vi "Get Last Plot Fit Data.vi"(8 "error in (no error)":errorcluster, 11 "XYGraph in":refnum<vi>) -> (0 "error out":errorcluster, 3 "Last Fit Data":T1)   [LabVIEW 2019, in "Histogram Window.lvlib"]
uses:
  Histogram Window.lvlib
  Plot Histogram.ctl
  Graphs/Plot Style 3.ctl
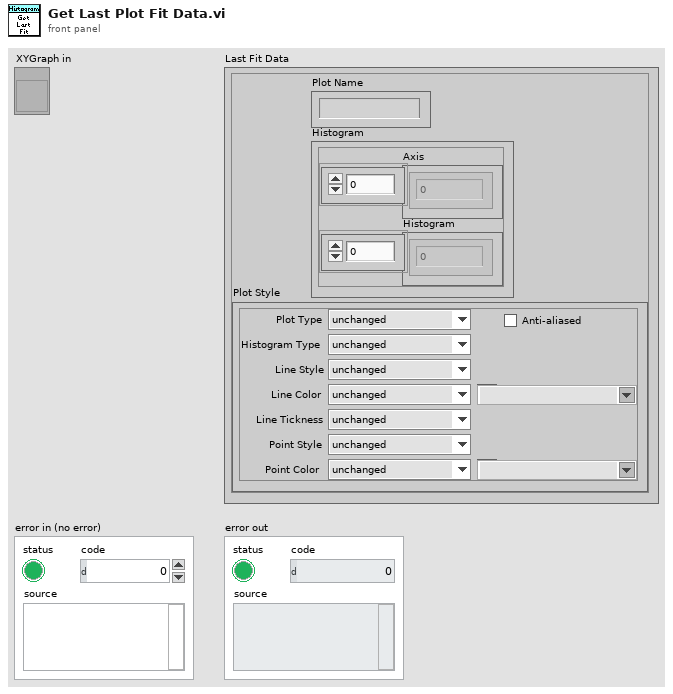
[diagram p1: front panel]
types:
  T1 = typedef "Histogram Window.lvlib/Plot Histogram.ctl" = cluster{"Plot Name":string, "Histogram":cluster{"Axis":dbl[], "Histogram":dbl[]}, "Plot Style":T2}
  T2 = typedef "Plot Style 3.ctl" = cluster{"Plot Style":enum16{"unchanged", "Line", "Symbol", "Line + Symbol", "Histogram", "Histogram + Symbol"}, "Histogram Type":enum16{"unchanged", "Left Bound", "Center", "Right Bound"}, "Line Tickness":enum16{"unchanged", "Thin", "1 pixel", "2 pixel", "3 pixel", "4 pixel", "5 pixel"}, "Line Style":enum16{"unchanged", "Plain", "Long Dash", "Short Dash", "Long-Short Dash", "Long-Short-Short Dash"}, "Point Style":enum16{"unchanged", "None", "Empty Circle", "Filled Circle", "Thick Circle", "Dotted Circle", "Empty Square", "Filled Square", "Thick Square", "Dotted Square", "Small Filled Square", "Dot", "Cross", "Tiny Cross", "Large X", "Small x", "Diamond", "Small Empty Square"}, "Line Color":u32, "Point Color":u32, "Anti-aliased":bool, "Line Color Chooser":enum16{"unchanged", "Color Box", "Color List"}, "Point Color Chooser":enum16{"unchanged", "Color Box", "Color List"}, "Line Color List":string, "Point Color List":string}
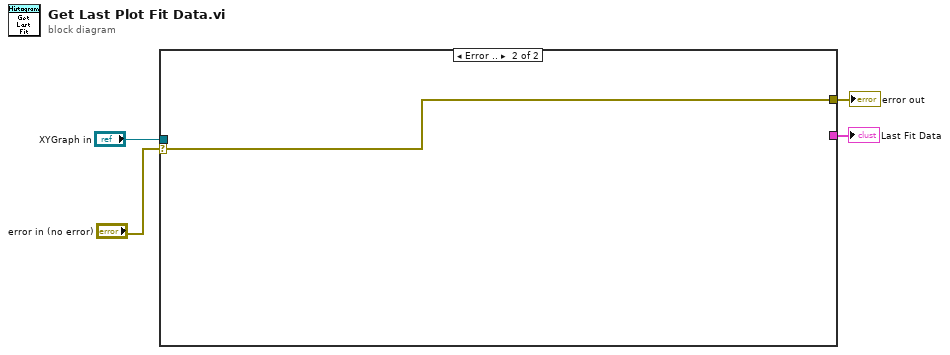
[diagram p0: block diagram]
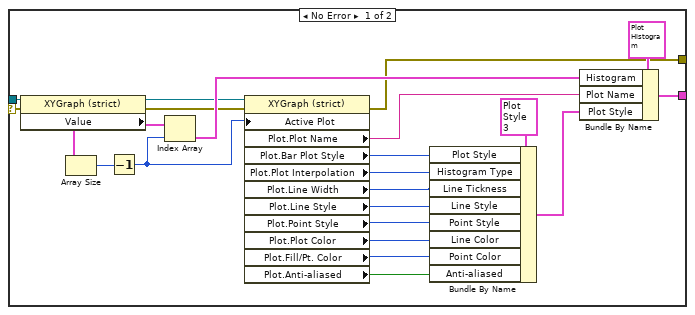
[diagram p2: hidden frame]
diagram:
  n1 = case shown="Error .." "error in (no error)" {
    selector: "error in (no error)" -> [w23 w27]
    tunnel: [w26 _] -> w4
    tunnel: "XYGraph in" -> [w24 _]
    tunnel: [w5 w27] -> w1
    frame No Error {
      n2 = property class="XYGraph (strict)"(reference=w24, error in=w23) -> (reference out=w19:refnum<vi>, error out=w18:errorcluster, "Value"=w22:cluster{"Axis":dbl[], "Histogram":dbl[]}[])
      n3 = Array Size(array=w22) -> (size(s)=w21:i32)
      n4 = Decrement(x=w21) -> (x-1=w17:i32)
      n5 = Index Array(array=w22, index=w17) -> (element=w20:cluster{"Axis":dbl[], "Histogram":dbl[]})
      n6 = property class="XYGraph (strict)"(reference=w19, error in=w18, "Active Plot"=w17) -> (error out=w5:errorcluster, "Plot.Plot Name"=w16:string, "Plot.Bar Plot Style"=w13:u8, "Plot.Plot Interpolation"=w14:u8, "Plot.Line Width"=w12:u8, "Plot.Line Style"=w11:u8, "Plot.Point Style"=w10:u8, "Plot.Plot Color"=w9:u32, "Plot.Fill/Pt. Color"=w8:u32, "Plot.Anti-aliased"=w7:bool)  [unwired: 1 out]
      n7 = Bundle By Name(cluster=T2 {"Plot Style"=enum."unchanged", "Histogram Type"=enum."Left Bound", "Line Tickness"=enum."unchanged", "Line Style"=enum."unchanged", "Point Style"=enum."unchanged", "Line Color"=0, "Point Color"=0, "Anti-aliased"=FALSE, "Line Color Chooser"=enum."unchanged", "Point Color Chooser"=enum."unchanged", "Line Color List"="", "Point Color List"=""} ("Plot Style"), "Plot Style"=w13, "Histogram Type"=w14, "Line Tickness"=w12, "Line Style"=w11, "Point Style"=w10, "Line Color"=w9, "Point Color"=w8, "Anti-aliased"=w7) -> (w6:T2)
      n8 = Bundle By Name(cluster=T1 {"Plot Name"="", "Histogram"={"Axis"=[], "Histogram"=[]}, "Plot Style"={"Plot Style"=enum."Line", "Histogram Type"=enum."Center", "Line Tickness"=enum."2 pixel", "Line Style"=enum."Plain", "Point Style"=enum."None", "Line Color"=16711680, "Point Color"=16711680, "Anti-aliased"=TRUE, "Line Color Chooser"=enum."Color Box", "Point Color Chooser"=enum."Color Box", "Line Color List"="", "Point Color List"=""}} ("output cluster"), "Histogram"=w20, "Plot Name"=w16, "Plot Style"=w6) -> (w26:T1)
    }
    frame Error {
    }
  }
  "error out" <- w1
  "Last Fit Data" <- w4
